vi "Periodic Tasks.vi"(8 "error in (no error)":errorcluster) -> ()   [LabVIEW 2013]
doc: "This VI runs in parallel to other tasks. It can contain as many user-defined periodic loops as you need. These can carry out PID or other sorts of timed response."
uses:
  <vilib>/Rock Robotics/SystemInterfaces/AI/FPGA_AIGyroChannel.ctl
  <vilib>/Rock Robotics/SystemInterfaces/Typedef/FPGA_TypedefAnalogModuleForGyro.ctl
  Example_Code/2014 Target Detection/TargetType.ctl
  TankDriveAction.ctl
  PnuematicMode.ctl
  QueueAction.ctl
  <vilib>/Rock Robotics/SystemInterfaces/Utilities/FPGA_UtilitiesLED Source.ctl
  <vilib>/Rock Robotics/SystemInterfaces/Utilities/FPGA_UtilitiesLED State.ctl
  Robot Global Data.vi
  <vilib>/Rock Robotics/WPI/Compressor/WPI_CompressorGetSetRefNum.vi
panel:
  in  "Color System":u16(ring)=2 items=["RGB", "HSL", "HSV", "HSI"]
  in  "Color Components":T1={"Hue"={116.0, 148.0}, "Sat"={152.0, 255.0}, "Val"={237.0, 255.0}} {"Val" scale=0.0..255.0; "Sat" scale=0.0..255.0; "Hue" scale=0.0..255.0 scale format="%#_3g"}
  out "Scores.State":T2
  out "Distance (ft)":dbl
  in  "Score cutoff":dbl=50.0
  out "Loop time (ms)":u32=51
  out "Angular Rate":dbl=0.1773163310546875
  in  "Analog Module":T3
  in  "Gain (VoltsPerDegree/Second)":dbl=0.007
  in  "Channel":T4
  in  "Reset Zero Position":bool
  out "Angle":dbl(knob)=4.4377348274728 scale=0.0..360.0
  out "error out":errorcluster
  # "GYRO"
  # "CAMERA"
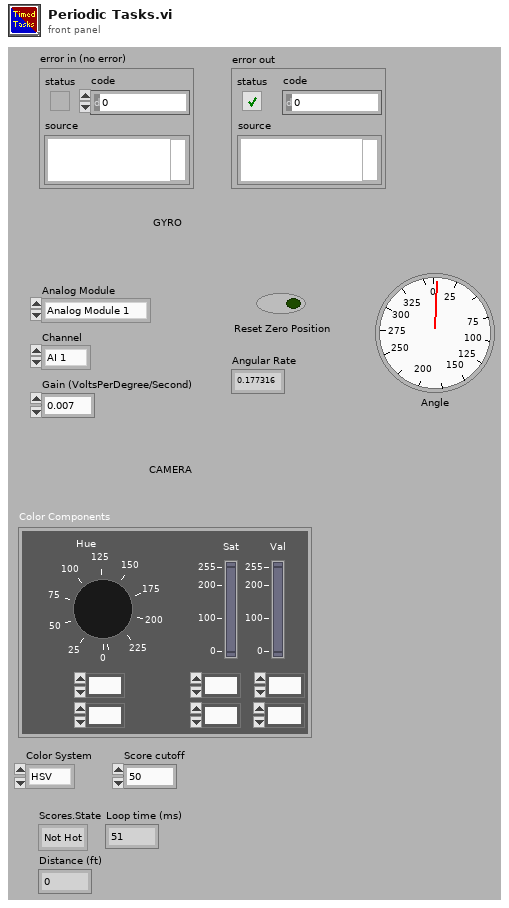
[diagram p1: front panel]
types:
  T1 = cluster{"Hue":cluster{dbl, dbl}, "Sat":cluster{dbl, dbl}, "Val":cluster{dbl, dbl}}
  T2 = typedef "TargetType.ctl" = enum16{"Not Hot", "Hot"}
  T3 = typedef "FPGA_TypedefAnalogModuleForGyro.ctl" = enum16{"Analog Module 1"}
  T4 = typedef "FPGA_AIGyroChannel.ctl" = enum8{"AI 1", "AI 2", "Invalid"}
  T5 = typedef "Image Type" = u32
  T6 = typedef "WPI_EncoderDevRef.ctl" = cluster{"DevStatus":errorcluster, "EncoderIndex":T7, "CounterIndex":T8, "DistancePerCount":dbl, "Decoding Type":T9}
  T7 = typedef "FPGA_EncoderIdx.ctl" = enum8{"Enc 0", "Enc 1", "Enc 2", "Enc 3", "Invalid"}
  T8 = typedef "FPGA_CounterCtrSystemIndex.ctl" = enum8{"Ctr 0", "Ctr 1", "Ctr 2", "Ctr 3", "Ctr 4", "Ctr 5", "Ctr 6", "Ctr 7", "Invalid"}
  T9 = typedef "WPI_EncoderType.ctl" = enum16{"1x", "2x", "4x"}
  T10 = typedef "WPI_GyroDevRef.ctl" = cluster{"DevStatus":errorcluster, "Analog Module":T11, "Analog Channel":T12, "Offset":dbl, "Gain (VoltsPerDegree/Second)":dbl}
  T11 = typedef "FPGA_TypedefAnalogModule.ctl" = enum16{"Analog Module 1", "Analog Module 2"}
  T12 = typedef "FPGA_AIChannel.ctl" = enum8{"AI 1", "AI 2", "AI 3", "AI 4", "AI 5", "AI 6", "AI 7", "AI 8", "Invalid"}
  T13 = typedef "WPI_SolenoidDevRef.ctl" = cluster{"DevStatus":errorcluster, "Solenoid Module":T14, "Forward Solenoid Channel":T15, "Reverse Solenoid Channel":T15}
  T14 = typedef "FPGA_TypedefSolenoidModule.ctl" = enum16{"Solenoid Module 1", "Solenoid Module 2"}
  T15 = typedef "WPI_SolenoidChannel.ctl" = enum8{"Solenoid 1", "Solenoid 2", "Solenoid 3", "Solenoid 4", "Solenoid 5", "Solenoid 6", "Solenoid 7", "Solenoid 8", "Invalid"}
  T16 = typedef "WPI_CameraDevRef.ctl" = cluster{"Camera Address":string, "CameraStatus":errorcluster, "Acquire Image Notifier":refnum<notifier>}
  T17 = typedef "IMAQ Image.ctl" = refnum<image>
  T18 = typedef "QueueAction.ctl" = enum16{"Init", "Get"}
  T19 = typedef "WPI_CameraImageSize.ctl" = enum16{"640x480", "320x240", "160x120"}
  T20 = typedef "TankDriveAction.ctl" = enum16{"Init", "LinearDrive", "SetValue", "Disable"}
  T21 = typedef "WPI_CompressorDevRef.ctl" = cluster{"DevStatus":errorcluster, "DigitalInputDevRef":T22, "RelayDevRef":T25}
  T22 = typedef "WPI_DigitalInputDevRef.ctl" = cluster{"DevStatus":errorcluster, "DIO Channel":T23, "Digital Module":T24}
  T23 = typedef "FPGA_DIOChannel.ctl" = enum8{"DIO 1", "DIO 2", "DIO 3", "DIO 4", "DIO 5", "DIO 6", "DIO 7", "DIO 8", "DIO 9", "DIO 10", "DIO 11", "DIO 12", "DIO 13", "DIO 14", "Invalid"}
  T24 = typedef "FPGA_TypedefDigitalModule.ctl" = enum16{"Digital Module 1", "Digital Module 2"}
  T25 = typedef "WPI_RelayDevRef.ctl" = cluster{"DevStatus":errorcluster, "Relay Channel":T26, "Digital Module":T24, "Relay Direction":T27}
  T26 = typedef "FPGA_DIORelayChannel.ctl" = enum8{"Relay 1", "Relay 2", "Relay 3", "Relay 4", "Relay 5", "Relay 6", "Relay 7", "Relay 8", "Invalid"}
  T27 = typedef "WPI_RelayDirection.ctl" = enum16{"Both directions", "Forward only", "Reverse only"}
  T28 = typedef "PnuematicMode.ctl" = enum16{"Init", "SetState", "Disable"}
  T29 = typedef "FPGA_UtilitiesLED State.ctl" = enum16{"Off", "On", "Toggle"}
  T30 = typedef "FPGA_UtilitiesLED Source.ctl" = enum16{"User LED", "FPGA LED"}
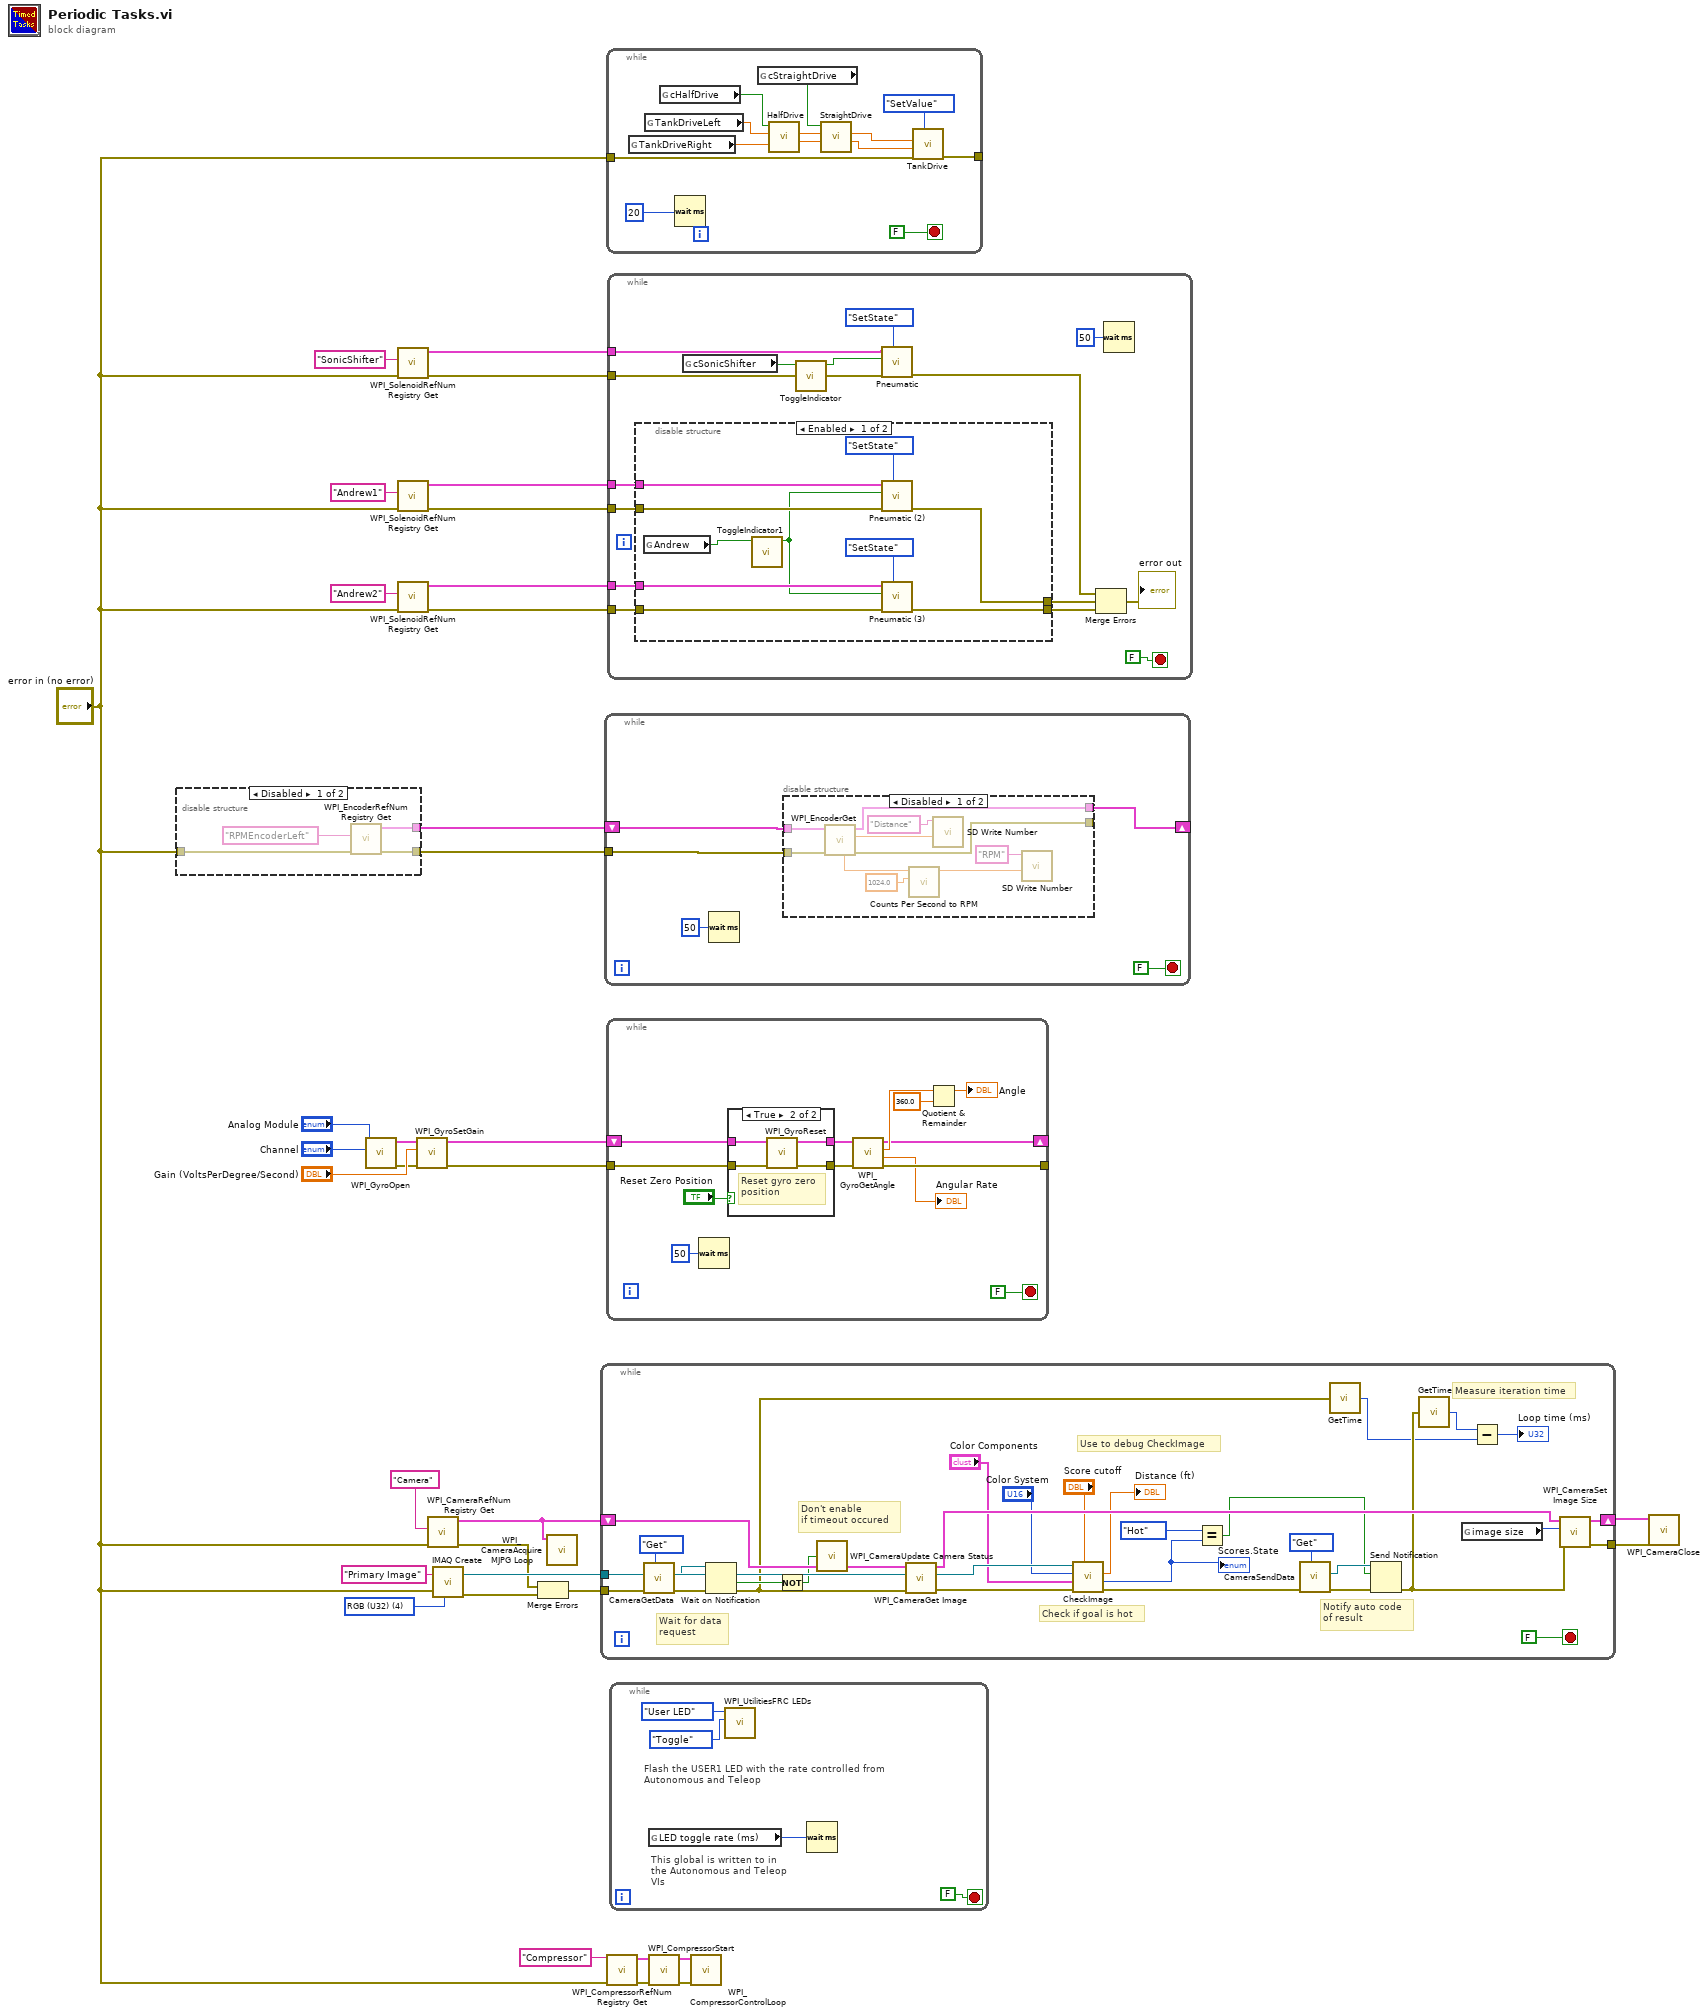
[diagram p0: block diagram]
diagram:
  w11 = T5 4 items=["Grayscale (U8)", "Grayscale (I16)", "Grayscale (SGL)", "Complex (CSG)", "RGB (U32)", "HSL (U32)", "RGB (U64)"] ("Image Type")
  n1 = disable-structure shown="Disabled" {
    disable-tunnel: [w37 _] -> w20
    disable-tunnel: [w36 _] -> w19
    disable-tunnel: "error in (no error)" -> [w35 _]
    frame Disabled {
      n2 = call <vilib>:"WPI_EncoderRefNum Registry Get.vi"("error in (no error)"=w35, "refnum name"="RPMEncoderLeft") -> ("error out"=w36:errorcluster, "EncoderDevRef"=w37:T6)  [unwired: 8 in]
    }
    frame Enabled {
    }
  }
  n3 = call <vilib>:"WPI_GyroOpen.vi"("Analog Channel"="Channel", "Analog Module (Module 1)"="Analog Module") -> ("error out"=w13:errorcluster, "GyroDevRef"=w17:T10)  [unwired: 4 in, 4 out]
  n4 = call <vilib>:"WPI_SolenoidRefNum Registry Get.vi"("error in (no error)"="error in (no error)", "refnum name"="SonicShifter") -> ("error out"=w27:errorcluster, "SolenoidDevRef"=w29:T13)  [unwired: 8 in]
  n5 = call <vilib>:"WPI_SolenoidRefNum Registry Get.vi"("error in (no error)"="error in (no error)", "refnum name"="Andrew1") -> ("error out"=w22:errorcluster, "SolenoidDevRef"=w24:T13)  [unwired: 8 in]
  n6 = call <vilib>:"WPI_SolenoidRefNum Registry Get.vi"("error in (no error)"="error in (no error)", "refnum name"="Andrew2") -> ("error out"=w21:errorcluster, "SolenoidDevRef"=w23:T13)  [unwired: 8 in]
  n7 = call <vilib>:"WPI_GyroSetGain.vi"("error in (no error)"=w13, "Gain (VoltsPerDegree/Second)"="Gain (VoltsPerDegree/Second)", "GyroDevRef"=w17) -> ("error out"=w12:errorcluster, "GyroDevRef"=w16:T10)  [unwired: 7 out]
  n8 = call <vilib>:"WPI_CameraRefNum Registry Get.vi"("error in (no error)"="error in (no error)", "refnum name"="Camera") -> ("error out"=w2:errorcluster, "CameraDevRef"=w7:T16)  [unwired: 8 in]
  n9 = call "IMAQ Create"("Image Name"="Primary Image", "Image Type"=w11, "error in (no error)"="error in (no error)") -> ("New Image"=w9:T17, "error out"=w1:errorcluster)  [unwired: 1 in, 1 out]
  n10 = Merge Errors(w2, w1) -> (w3:errorcluster)
  n11 = call <vilib>:"WPI_CameraAcquire MJPG Loop.vi"("CameraDevRef"=w7) -> ()  [unwired: 11 in]
  n12 = while {
    shift-right: [w69] -> w5
    shift-left: w7 -> [w67]
    tunnel: w9 -> [w68]
    tunnel: w3 -> [w55]
    tunnel: [w45] -> w4
    stop <- FALSE stop-if-true
    # "Wait for data\nrequest"
    # "Use to debug CheckImage"
    # "Check if goal is hot"
    # "Notify auto code\nof result"
    # "Measure iteration time"
    # "Don't enable\nif timeout occured"
    n13 = call "CameraGetData.vi"("Action"=QueueAction."Get", "error in"=w55) -> ("error out"=w54:errorcluster, "notifier out"=w53:refnum<notifier>)  [unwired: 8 in]
    n14 = Wait on Notification(notifier=w53, error in (no error)=w54) -> (timed out?=w51:bool, error out=w44:errorcluster)  [unwired: 2 in, 2 out]
    n15 = Not(x=w51) -> (.not. x?=w52:bool)
    n16 = call <vilib>:"WPI_CameraUpdate Camera Status.vi"("CameraDevRef In"=w67, "Enable Vision"=w52) -> ("CameraDevRef Out"=w66:T16)  [unwired: 3 in]
    n17 = call <vilib>:"WPI_CameraGet Image.vi"("error in (no error)"=w44, "Image"=w68, "CameraDevRef"=w66) -> ("error out"=w50:errorcluster, "Image Out"=w62:T17, "CameraDevRef Out"=w63:T16)  [unwired: 6 out]
    n18 = call "CheckImage.vi"("Score cutoff"="Score cutoff", "error in"=w50, "Color Components"="Color Components", "Color System"="Color System", "Image"=w62) -> ("error out"=w49:errorcluster, "Scores.State"=w56:T2, "Distance (ft)"=→"Distance (ft)":dbl)  [unwired: 3 in, 1 out]
    "Scores.State" <- w56
    n19 = Equal?(x=TargetType."Hot" ("Scores.State 2"), y=w56) -> (x = y?=w46:bool)
    n20 = call "CameraSendData.vi"("Action"=QueueAction."Get", "error in"=w49) -> ("error out"=w48:errorcluster, "notifier out"=w47:refnum<notifier>)  [unwired: 8 in]
    n21 = call "GetTime.vi"("error in"=w44) -> ("Time"=w42:u32)
    n22 = Send Notification(notification=w46, notifier=w47, error in (no error)=w48) -> (error out=w43:errorcluster)  [unwired: 1 out]
    n23 = call "GetTime.vi"("error in"=w43) -> ("Time"=w41:u32)
    n24 = global read "Robot Global Data.vi" "image size"() -> (w64:T19)
    n25 = Subtract(x=w41, y=w42) -> (x-y=→"Loop time (ms)":u32)
    n26 = call <vilib>:"WPI_CameraSet Image Size.vi"("error in (no error)"=w43, "Image Size"=w64, "CameraDevRef"=w63) -> ("error out"=w45:errorcluster, "CameraDevRef Out"=w69:T16)  [unwired: 7 out]
  }
  n27 = while {
    tunnel: w19 -> [w72]
    shift-right: [w71] -> _
    shift-left: w20 -> [w73]
    stop <- FALSE stop-if-true
    n28 = Wait (ms)(milliseconds to wait=u32 50) -> ()  [unwired: 1 out]
    n29 = disable-structure shown="Disabled" {
      disable-tunnel: w72 -> [w85 _]
      disable-tunnel: w73 -> [w78 _]
      disable-tunnel: [w77 _] -> _
      disable-tunnel: [w76 _] -> w71
      frame Disabled {
        n30 = call <vilib>:"WPI_EncoderGet.vi"("error in (no error)"=w85, "EncoderDevRef"=w78) -> ("error out"=w77:errorcluster, "Distance"=w80:dbl, "EncoderDevRef"=w76:T6, "Rate"=w84:dbl)  [unwired: 4 in, 2 out]
        n31 = call "Counts Per Second to RPM.vi"("Counts/Rev"=1024.0, "Counts/Second"=w84) -> ("RPM"=w82:dbl)  [unwired: 9 in]
        n32 = call <vilib>:"SD Write Number.vi"("Numeric"=w80, "Name"="Distance") -> ()  [unwired: 8 in, 2 out]
        n33 = call <vilib>:"SD Write Number.vi"("Numeric"=w82, "Name"="RPM") -> ()  [unwired: 8 in, 2 out]
      }
      frame Enabled {
      }
    }
  }
  n34 = while {
    tunnel: "error in (no error)" -> [w95]
    tunnel: [w94] -> _
    stop <- FALSE stop-if-true
    n35 = global read "Robot Global Data.vi" "TankDriveRight"() -> (w88:dbl)
    n36 = global read "Robot Global Data.vi" "TankDriveLeft"() -> (w89:dbl)
    n37 = global read "Robot Global Data.vi" "cHalfDrive"() -> (w87:bool)
    n38 = Wait (ms)(milliseconds to wait=u32 20) -> ()  [unwired: 1 out]
    n39 = global read "Robot Global Data.vi" "cStraightDrive"() -> (w86:bool)
    n40 = call "HalfDrive.vi"("RightDrive in"=w88, "LeftDrive in"=w89, "HalfDrive"=w87) -> ("RightDrive out"=w92:dbl, "LeftDrive out"=w93:dbl)  [unwired: 7 in]
    n41 = call "StraightDrive.vi"("RightDrive in"=w92, "LeftDrive in"=w93, "StraightDrive"=w86) -> ("RightDrive out"=w90:dbl, "LeftDrive out"=w91:dbl)  [unwired: 7 in]
    n42 = call "TankDrive.vi"("DriveAction"=TankDriveAction."SetValue" ("Enum"), "error in (no error)"=w95, "RightDesired"=w90, "LeftDesired"=w91) -> ("error out"=w94:errorcluster)  [unwired: 7 in]
  }
  n43 = while {
    shift-right: [w107] -> _
    shift-left: w16 -> [w110]
    tunnel: w12 -> [w103]
    tunnel: [w101] -> _
    stop <- FALSE stop-if-true
    n44 = Wait (ms)(milliseconds to wait=u32 50) -> ()  [unwired: 1 out]
    n45 = case shown="True" "Reset Zero Position" {
      tunnel: w110 -> [w112 w116]
      tunnel: [w112 w115] -> w109
      tunnel: w103 -> [_ w114]
      tunnel: [_ w113] -> w102
      frame False {
      }
      frame True {
        # "Reset gyro zero \nposition"
        n46 = call <vilib>:"WPI_GyroReset.vi"("error in (no error)"=w114, "GyroDevRef"=w116) -> ("error out"=w113:errorcluster, "GyroDevRef"=w115:T10)  [unwired: 8 out]
      }
    }
    n47 = call <vilib>:"WPI_GyroGetAngle.vi"("error in (no error)"=w102, "GyroDevRef"=w109) -> ("error out"=w101:errorcluster, "Angular Rate"=→"Angular Rate":dbl, "Angle"=w108:dbl, "GyroDevRef"=w107:T10)  [unwired: 6 out]
    n48 = Quotient & Remainder(x=w108, y=360.0) -> (x-y*floor(x/y)=→"Angle":dbl)  [unwired: 1 out]
  }
  n49 = call <vilib>:"WPI_CompressorRefNum Registry Get.vi"("error in (no error)"="error in (no error)", "refnum name"="Compressor") -> ("error out"=w31:errorcluster, "CompressorDevRef"=w34:T21)  [unwired: 8 in]
  n50 = while {
    tunnel: w29 -> [w129]
    tunnel: w27 -> [w130]
    tunnel: w24 -> [w125]
    tunnel: w23 -> [w124]
    tunnel: w22 -> [w127]
    tunnel: w21 -> [w123]
    stop <- FALSE stop-if-true
    n51 = disable-structure shown="Enabled" {
      disable-tunnel: w127 -> [w141 _]
      disable-tunnel: [w140 _] -> w126
      disable-tunnel: w125 -> [w139 _]
      disable-tunnel: w124 -> [w137 _]
      disable-tunnel: w123 -> [w136 _]
      disable-tunnel: [w135 _] -> w122
      frame Enabled {
        n52 = global read "Robot Global Data.vi" "Andrew"() -> (w133:bool)
        n53 = call "ToggleIndicator1.vi"("cSonicShifter"=w133) -> ("Actuate?"=w132:bool)  [unwired: 10 in]
        n54 = call "Pneumatic (2).vi"("Mode"=PnuematicMode."SetState", "error in (no error)"=w141, "State"=w132, "SolenoidDevRef"=w139) -> ("error out"=w140:errorcluster)  [unwired: 7 in]
        n55 = call "Pneumatic (3).vi"("Mode"=PnuematicMode."SetState", "error in (no error)"=w136, "State"=w132, "SolenoidDevRef"=w137) -> ("error out"=w135:errorcluster)  [unwired: 7 in]
      }
      frame Disabled {
      }
    }
    n56 = global read "Robot Global Data.vi" "cSonicShifter"() -> (w121:bool)
    n57 = call "ToggleIndicator.vi"("cSonicShifter"=w121) -> ("Actuate?"=w120:bool)  [unwired: 10 in]
    n58 = call "Pneumatic.vi"("Mode"=PnuematicMode."SetState", "error in (no error)"=w130, "State"=w120, "SolenoidDevRef"=w129) -> ("error out"=w117:errorcluster)  [unwired: 7 in]
    n59 = Merge Errors(w117, w126, w122) -> (→"error out":errorcluster)
    n60 = Wait (ms)(milliseconds to wait=u32 50) -> ()  [unwired: 1 out]
  }
  n61 = while {
    stop <- FALSE stop-if-true
    # "This global is written to in the Autonomous and Teleop VIs"
    # "Flash the USER1 LED with the rate controlled from Autonomous and Teleop"
    n62 = global read "Robot Global Data.vi" "LED toggle rate (ms)"() -> (w142:u32)
    n63 = call <vilib>:"WPI_UtilitiesFRC LEDs.vi"("State"=FPGA_UtilitiesLED_State."Toggle", "LED Type"=FPGA_UtilitiesLED_Source."User LED") -> ()  [unwired: 1 in, 9 out]
    n64 = Wait (ms)(milliseconds to wait=w142) -> ()  [unwired: 1 out]
  }
  n65 = call <vilib>:"WPI_CompressorStart.vi"("error in (no error)"=w31, "CompressorDevRef"=w34) -> ("error out"=w28:errorcluster, "CompressorDevRef"=w33:T21)  [unwired: 8 in]
  n66 = call <vilib>:"WPI_CompressorControlLoop.vi"("error in (no error)"=w28, "CompressorDevRef"=w33) -> ()  [unwired: 10 in]
  n67 = call <vilib>:"WPI_CameraClose.vi"("error in (no error)"=w4, "CameraDevRef"=w5) -> ()  [unwired: 10 out]
